vi "UniPend - NonLinear Model.vi"(0 "initial alpha":dbl=3.1416, 1 "initial velocity alpha":dbl, 7 "Torque (Tau)":dbl=1.0, 12 "friction coefficient 1":dbl=0.02, 14 "Amplifier Gain":dbl(slide)=0.4 scale=0.0..3.0) -> (6 "alpha1":dbl=0.11676928692181643)   [LabVIEW 2012]
uses:
  <vilib>/Simulation/Implementation/Shared/SIMSCR Execution Mode.ctl
  <vilib>/Simulation/Scripting/Companion Diagram/SimConfigNode/SimParams.ctl
  <vilib>/Simulation/Scripting/Companion Diagram/SimConfigNode/_simSolvers.ctl
  <vilib>/Simulation/Param Hierarchy/Typedefs/SIMPH Param Control Actions.ctl
  <vilib>/Simulation/Implementation/Shared/SIM limit type.ctl
  <vilib>/Simulation/Implementation/Shared/NILVSim_ParamChanged.vi
  <vilib>/Simulation/ContinuousLinear/Implementation/NILVSim Integrator new.llb/SIM Integrator distributor (scalar).vi
  <vilib>/Simulation/ContinuousLinear/Implementation/NILVSim Integrator new.llb/SIM Integrator collector (scalar).vi
  <vilib>/Simulation/Implementation/Shared/NILVSim_Manager.vi
  <vilib>/Simulation/Implementation/Shared/NILVSim_FinalizeModel.vi
  <vilib>/Simulation/Implementation/Shared/SIM Unbundle Sim Info.vi
  <vilib>/Utility/error.llb/Clear Errors.vi
  <vilib>/Simulation/Implementation/Shared/NILVSim_GetModelError.vi
  <vilib>/Simulation/Implementation/Shared/SIM SimErrorHandler.vi
  <vilib>/Simulation/Implementation/Shared/SIM Bundle Sim Info.vi
  <vilib>/Simulation/Implementation/Shared/SIMSH Read Queue.vi
  <vilib>/Simulation/Implementation/Shared/NILVSim_Initialize.vi
  <vilib>/Simulation/Utility/Implementation/NILVSim Get Time and IsAcceptedStep.vi
  <vilib>/Simulation/Scripting/Companion Diagram/SimConfigNode/SimDog.xnode
  <vilib>/Simulation/Implementation/XNodeFramework/SimXNode/SimX.xnode
  <vilib>/Simulation/ContinuousLinear/Implementation/NILVSim Integrator new.llb/SIM Integrator (scalar).vi
  <vilib>/ptbypt/NI_PtbyPt.lvlib
  <vilib>/Simulation/Implementation/Shared/NI_SIM_Implementation.lvlib
panel:
  out "states":dbl[](array[numeric])=[0.11676928692181643, -0.3578561321200968, -0.19175807659191071, 0.3912657493379608]
  in  "Gravitational Force (m/s^2)":dbl=9.81
  in  "Moment of Inetia of the frame wrt to center of mass (Ifg)":dbl=20.0
  in  "Distance from center of wheel to center of mass (Rf)":dbl=0.463
  in  "Radius of Wheel (Rw)":dbl=0.2032
  in  "Moment of Inertia wrt center of mass (Iwg)":dbl=0.0812
  in  "Mass of Frame (mf)":dbl=25.0
  in  "Mass of Bottom Wheel (mw)":dbl=7.645
  # "Legend: \nC.G.  - Center of Gravity\nl       - Length (m)\nJ      - Moment of Inertia (kg(m^2)\nM     - Mass (kg)"
  # "Derived Parameters"
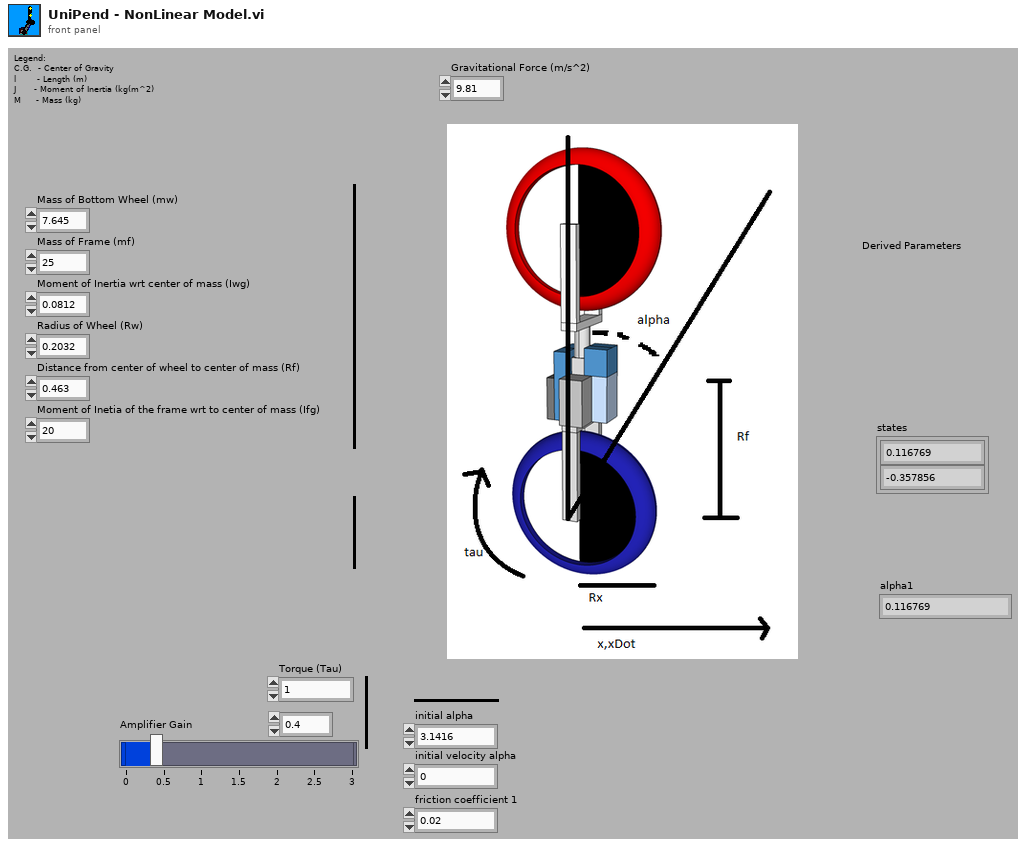
[diagram p1: front panel]
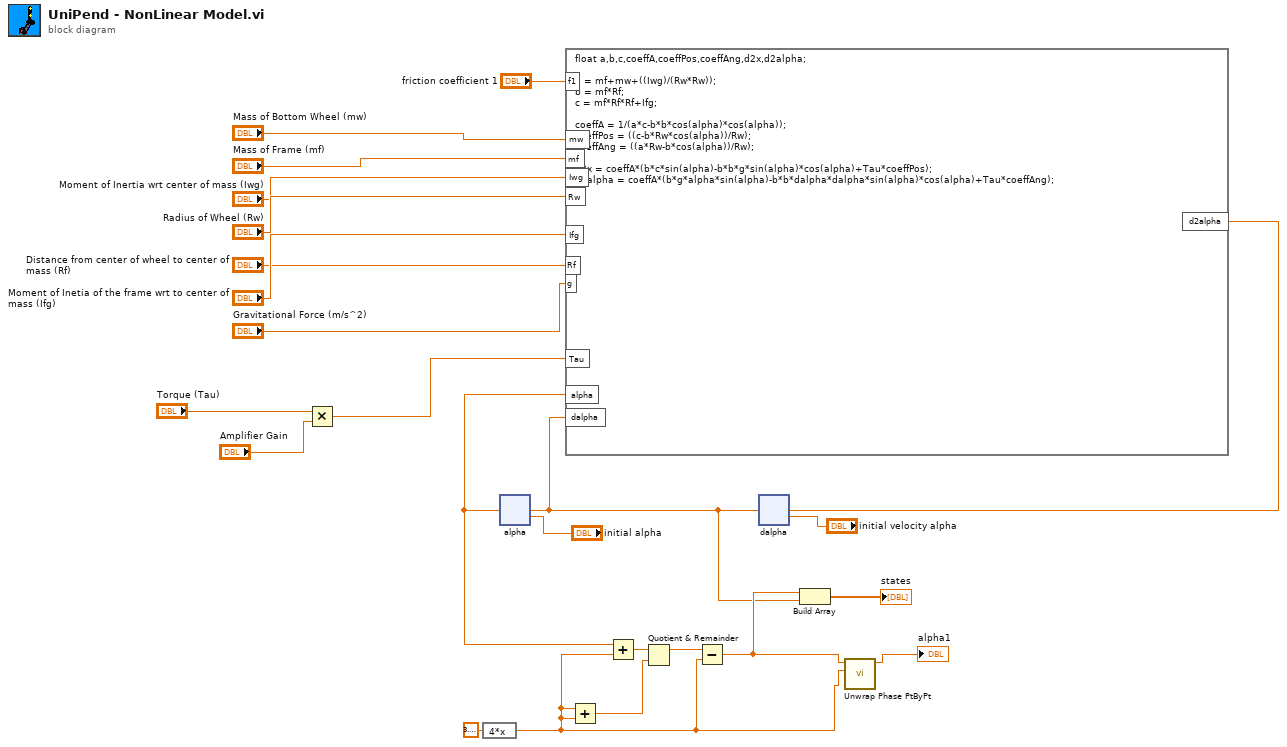
[diagram p0: block diagram]
diagram:
  n1 = Multiply ("Multiply 8")(x="Torque (Tau)", y="Amplifier Gain") -> (x*y=w22:dbl)
  n2 = expression code="4*x"(3.141592653589793 ("Constant")) -> (w11:dbl)
  n3 = Add ("Add 6")(x=w11, y=w11) -> (x+y=w13:dbl)
  n4 = xnode "alpha"("input"=w2, "initial condition"="initial alpha") -> ("output"=w15:dbl)  [unwired: 8 in, 2 out]
  n5 = Add ("Add 5")(x=w15, y=w11) -> (x+y=w16:dbl)
  n6 = Quotient & Remainder ("Quotient & Remainder 2")(x=w16, y=w13) -> (x-y*floor(x/y)=w17:dbl)  [unwired: 1 out]
  n7 = Subtract ("Subtract 2")(x=w17, y=w11) -> (x-y=w3:dbl)
  n8 = call <vilib>:"Unwrap Phase PtByPt.vi"("wrap base"=w11, "phase"=w3) -> ("unwrapped phase"=→"alpha1":dbl)  [unwired: 9 in]
  n9 = formula code="float a,b,c,coeffA,coeffPos,coeffAng,d2x,d2alpha;\n\na = mf+mw+((Iwg)/(Rw*Rw));\nb = mf*Rf;\nc = mf*Rf*Rf+Ifg;\n\ncoeffA = 1/(a*c-b*b*cos(alpha)*cos(alpha));\ncoeffPos = ((c-b*Rw*cos(alpha))/Rw);\ncoeffAng = ((a*Rw-b*cos(alpha))/Rw);\n\nd2x = coeffA*(b*c*sin(alpha)-b*b*g*sin(alpha)*cos(alpha)+Tau*coeffPos);\nd2alpha = coeffA*(b*g*alpha*sin(alpha)-b*b*dalpha*dalpha*sin(alpha)*cos(alpha)+Tau*coeffAng);"("Tau"=w22, "alpha"=w15, "dalpha"=w2, "f1"="friction coefficient 1", "mw"="Mass of Bottom Wheel (mw)", "mf"="Mass of Frame (mf)", "Iwg"="Moment of Inertia wrt center of mass (Iwg)", "Rw"="Radius of Wheel (Rw)", "Rf"="Distance from center of wheel to center of mass (Rf)", "Ifg"="Moment of Inetia of the frame wrt to center of mass (Ifg)", "g"="Gravitational Force (m/s^2)") -> ("d2alpha"=w24:dbl)
  n10 = xnode "dalpha"("input"=w24, "initial condition"="initial velocity alpha") -> ("output"=w2:dbl)  [unwired: 8 in, 2 out]
  n11 = Build Array(w3, w2) -> (→"states":dbl[])
